vi "Correlator port.vi"() -> ()   [LabVIEW 2012]
panel:
  in  "Addr (0-15)":i8 min=0 max=15 step=1
  in  "VISA resource name":refnum<visa-resource-name>="COM1"
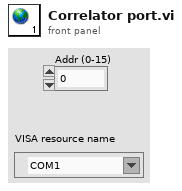
[diagram p1: front panel]
diagram:
